vi "PH_PILS.PC _DoorTags.vi"(0 "i ref in":refnum<vi>, 2 "serviceName":string, 3 "Value":i32, 5 "error IO":errorcluster) -> (14 "i ref out":refnum<vi>, 19 "error out":errorcluster)   [LabVIEW 2014, in "PH_PILS.lvlib"]
doc: "This VI writes the incoming information to owbn attributes."
uses:
  PH_PILS.lvlib
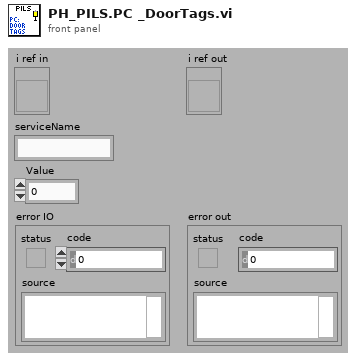
[diagram p1: front panel]
types:
  T1 = typedef "PH_PILS.lvlib/PH_PILS.i attribute.ctl" = cluster{"Boolean":cluster{"GUI Ref":refnum<vi>, "Status":i32}[], "GUI Refs Exp. Shutters":cluster{"1":refnum<vi>, "2":refnum<vi>, "3":refnum<vi>, "4":refnum<vi>}, "Tristate2Run GUI Refs":refnum<vi>[], "EO-Likes":cluster{"GUI Ref":refnum<vi>, "Status":i32}[], "Operation Mode":cluster{"Operation Mode":T2, "GUI":cluster{"Ref State":refnum<vi>, "Ref":refnum<vi>}, "Servicemode":cluster{"Tagname":string, "Status":i32}, "Labormode":cluster{"Tagname":string, "Status":i32}, "Searchmode":cluster{"Tagname":string, "Status":i32}, "Shotmode":cluster{"Tagname":string, "Status":i32}}, "Submode":cluster{"Submode":T3, "GUI":cluster{"Ref State":refnum<vi>, "Ref":refnum<vi>}, "Submode":cluster{"Tagname":string, "Status":i32}}, "Experiment":cluster{"Experiment":enum16{"unknown", "intern", "4 (Z6)", "3", "2", "1"}, "GUI":cluster{"Ref State":refnum<vi>, "Ref":refnum<vi>}, "intern":cluster{"Tagname":string, "Status":i32}, "Exp 4":cluster{"Tagname":string, "Status":i32}, "Exp 3":cluster{"Tagname":string, "Status":i32}, "Exp 2":cluster{"Tagname":string, "Status":i32}, "Exp 1":cluster{"Tagname":string, "Status":i32}}, "TristateNormal":cluster{"GUI Ref":refnum<vi>, "Status":i32}[], "Door Tags":cluster{"GUI Ref":refnum<vi>, "Status":i32}[], "GUIlessTags":cluster{"Name":string, "Status":i32}[], "Beamline GUI Refs":refnum<vi>[], "Special Boolean":cluster{"GUI Ref":refnum<vi>, "Status":i32}[], "Laserpower":cluster{"GUI Ref":refnum<vi>, "Status":i32}[], "Shutter":cluster{"GUI Ref":refnum<vi>, "Status":i32}[], "Tristate EO Like":cluster{"GUI Ref":refnum<vi>, "Status":i32}[], "PP":cluster{"GUI Ref":refnum<vi>, "Status":i32, "Head Ref":refnum<vi>, "Slider Ref":refnum<vi>}[], "Switch Knobs":cluster{"GUI Ref":refnum<vi>, "Status":i32}[], "Latch Knob GUI Refs":refnum<vi>[], "FailureCounter":i32, "Enabled Status":cluster{"Laser":i32, "PreAmp":i32, "MainAmp":i32}, "Mercury":refnum<vi>, "Instance Rods":string, "Logfile":path, "Beckhoff-Instance Internal":string, "Beckhoff-Instance External":string, "Enabling Rights":cluster{"Name":string, "Password":string, "PA?":bool, "MA?":bool, "Exp?":bool}[]}
  T2 = typedef "PH_PILS.lvlib/PH_PILS.Operation Mode.ctl" = enum16{"unknown", "Service", "Labor", "Search", "Shot"}
  T3 = typedef "PH_PILS.lvlib/PH_PILS.Submode.ctl" = enum16{"unknown", "HV-Normal", "HV-Test"}
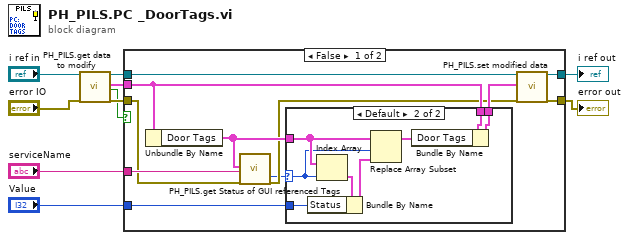
[diagram p0: block diagram]
diagram:
  n1 = call "PH_PILS.get data to modify.vi"("i ref in"="i ref in", "error in (no error)"="error IO") -> ("i ref out"=w5:refnum<vi>, "i attribute"=w6:T1, "timed out"=w2:bool, "error out"=w7:errorcluster)  [unwired: 14 in]
  n2 = case shown="False" w2 {
    tunnel: "Value" -> [w16 _]
    tunnel: "serviceName" -> [w14 _]
    tunnel: w7 -> [w13 w31]
    tunnel: w6 -> [w18 _]
    tunnel: w5 -> [w21 w32]
    tunnel: [w20 w32] -> w4
    tunnel: [w19 w31] -> w3
    frame False {
      n3 = Unbundle By Name(w18) -> ("Door Tags"=w15:cluster{"GUI Ref":refnum<vi>, "Status":i32}[])
      n4 = call "PH_PILS.get Status of GUI referenced Tags.vi"("Tags"=w15, "Tagname"=w14, "error in"=w13) -> ("index of element"=w11:i32, "error out"=w12:errorcluster)  [unwired: 13 in, 2 out]
      n5 = case shown="Default" w11 {
        selector: w11 -> [_ w23]
        tunnel: w15 -> [_ w30]
        tunnel: w18 -> [w22 w29]
        tunnel: [w22 w28] -> w17
        tunnel: w16 -> [_ w24]
        frame -1 {
        }
        frame Default {
          n6 = Index Array(array=w30, index=w23) -> (element=w26:cluster{"GUI Ref":refnum<vi>, "Status":i32})
          n7 = Bundle By Name(cluster=w26, "Status"=w24) -> (w25:cluster{"GUI Ref":refnum<vi>, "Status":i32})
          n8 = Replace Array Subset(array=w30, new element=w25, index=w23) -> (w27:cluster{"GUI Ref":refnum<vi>, "Status":i32}[])
          n9 = Bundle By Name(cluster=w29, "Door Tags"=w27) -> (w28:T1)
        }
      }
      n10 = call "PH_PILS.set modified data.vi"("i ref in"=w21, "i attribute"=w17, "error in (no error)"=w12) -> ("i ref out"=w20:refnum<vi>, "error out"=w19:errorcluster)  [unwired: 15 in]
    }
    frame True {
    }
  }
  "error out" <- w3
  "i ref out" <- w4
